vi "Ponk.vi"() -> ()   [LabVIEW 2022 SP3]
uses:
  <vilib>/Utility/miscctls.llb/LVPositionTypeDef.ctl
panel:
  out "BarPosition 2":T1
  out "Bar 2":bool
  out "Top":bool
  out "exit?":bool
  in  "STOP":bool
  out "BarPosition":T1
  out "BallPosition":T1
  out "Step":T1
  out "Bar":bool
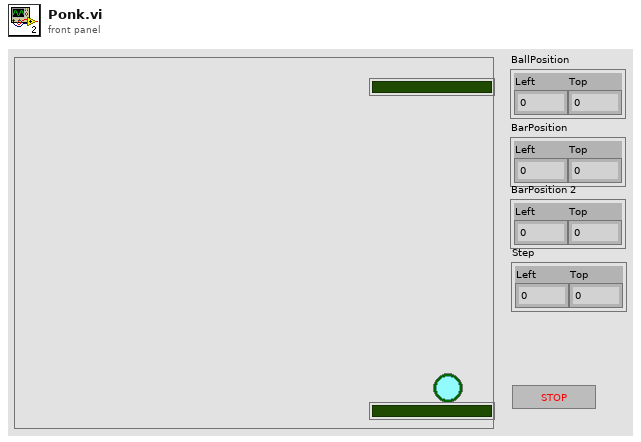
[diagram p1: front panel]
types:
  T1 = typedef "LVPositionTypeDef.ctl" = cluster{"Left":i32, "Top":i32}
  T2 = cluster{"BallPosition":T1, "Step":T1, "Score":i32, "BarPosition":T1, "BarPosition_2":T1}
  T3 = typedef "LVBoundsTypeDef.ctl" = cluster{"Width":u32, "Height":u32}
  T4 = typedef "eventvkey.ctl" = enum16{"ASCII", "Enter", "Return", "Shift", "Ctrl", "Alt", "Cmd", "Opt", "Caps", "NumLock", "Clear", "Break", "Up", "Down", "Left", "Right", "Insert", "Delete", "Home", "End", "PageUp", "PageDown", "Escape", "Help", "Pause", "ScrollLock", "F1", "F2", "F3", "F4", "F5", "F6", "F7", "F8", "F9", "F10", "F11", "F12", "F13", "F14", "F15", "F16", "F17", "F18", "F19", "F20", "F21", "F22", "F23", "F24", "Play", "VolumeUp", "VolumeDown", "Mute", "Two Byte Char"}
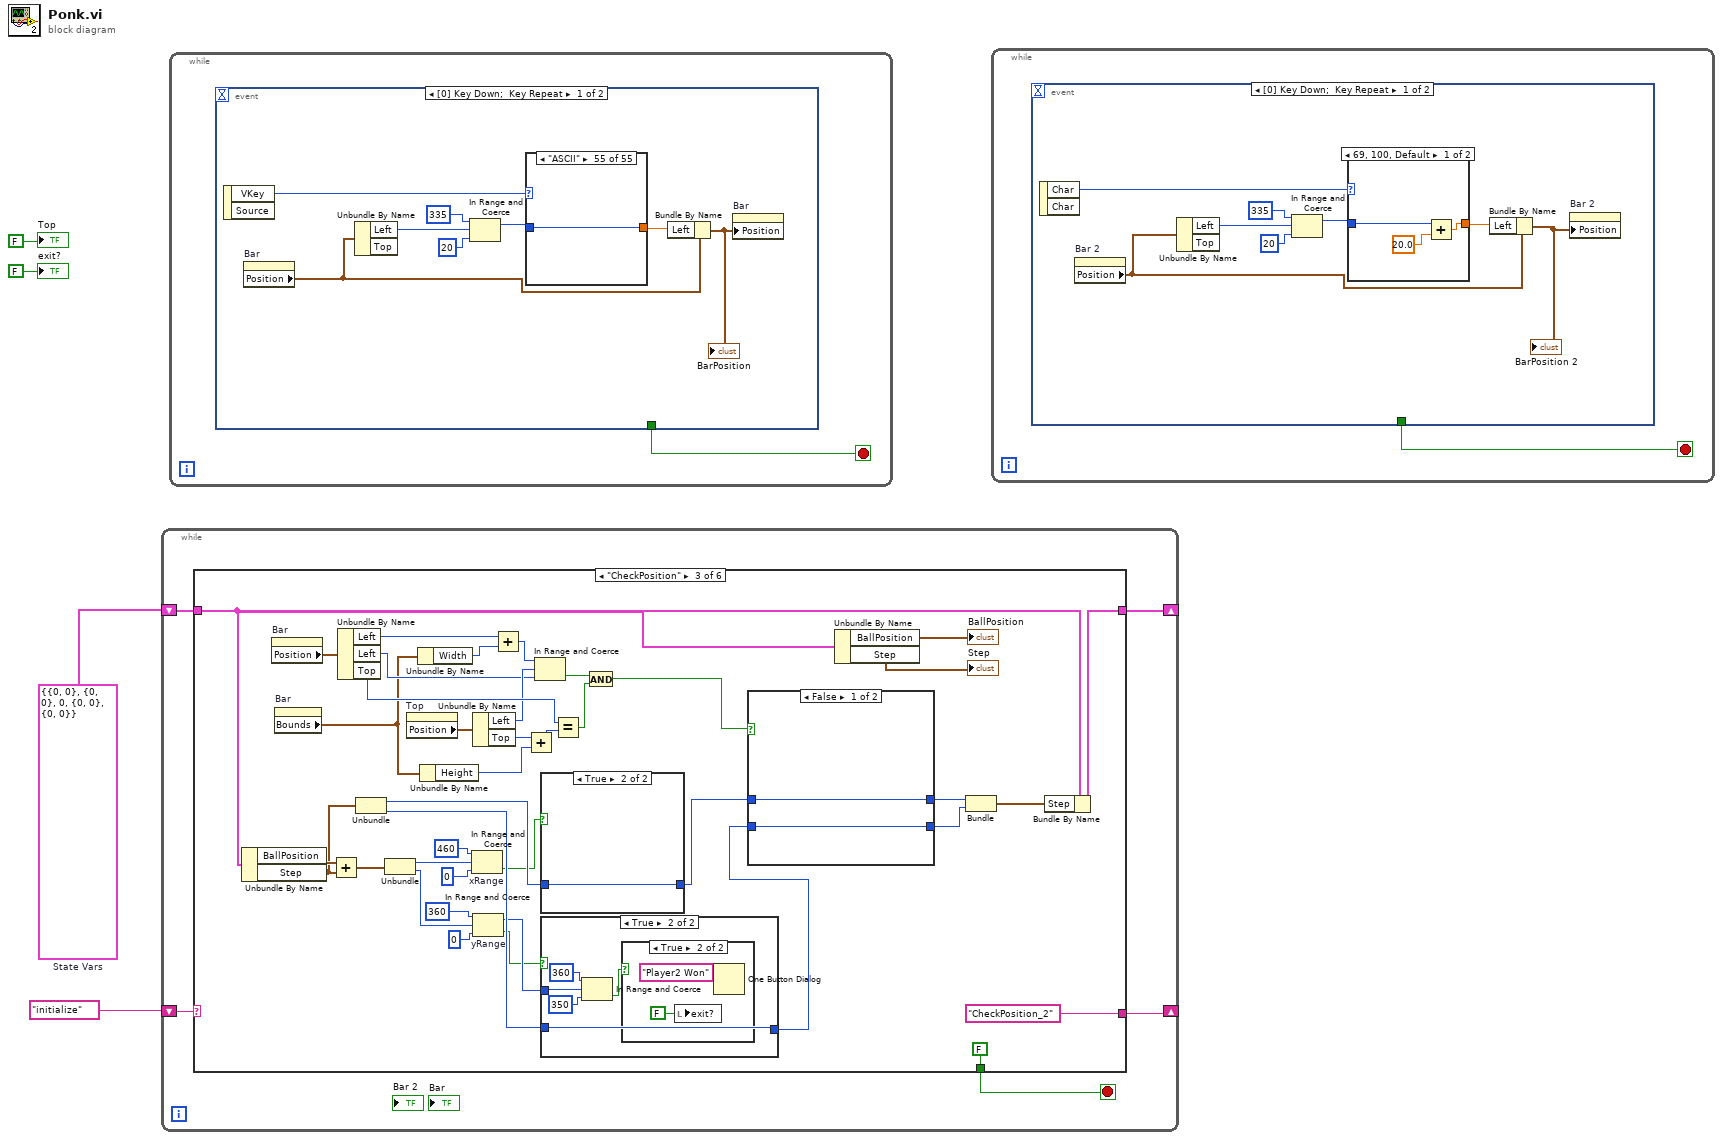
[diagram p0: block diagram]
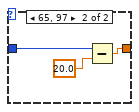
[diagram p2: hidden frame]
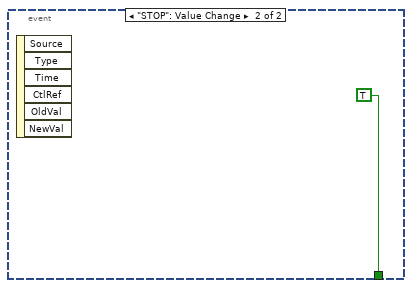
[diagram p3: hidden frame]
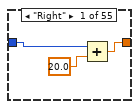
[diagram p4: hidden frame]
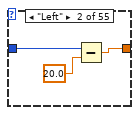
[diagram p5: hidden frame]
diagram:
  w3 = T2 {"BallPosition"={"Left"=0, "Top"=0}, "Step"={"Left"=0, "Top"=0}, "Score"=0, "BarPosition"={"Left"=0, "Top"=0}, "BarPosition_2"={"Left"=0, "Top"=0}}  # State Vars
  n1 = while {
    shift-right: [w7] -> _
    shift-left: "initialize" -> [w6]
    shift-right: [w8] -> _
    shift-left: w3 -> [w9]
    stop <- w5 stop-if-true
    n2 = case shown="\"CheckPosition\"" w6 {
      selector: w6 -> [w11 _ _ _ _ _]
      tunnel: w9 -> [w12 w30 w43 w99 w144 w147]
      tunnel: [w12 w29 w60 w115 w144 w151] -> w8
      tunnel: [w11 "UpdateBallPosition" "CheckPosition_2" "Stop" "UpdateBallPosition" "CheckPosition"] -> w7
      tunnel: [FALSE ("STOP") FALSE ("STOP") FALSE ("STOP") FALSE ("STOP") "STOP" FALSE ("STOP")] -> w5
      frame "False", Default {
      }
      frame "Initialize" {
        n3 = property on="Bar" class="Bool (strict)"() -> ("Bounds"=w23:T3)  [unwired: 2 in, 2 out]
        n4 = Unbundle By Name(w23) -> ("Width"=w22:u32)
        n5 = property on="Bar" class="Bool (strict)"() -> ("Position"=w24:T1)  [unwired: 2 in, 2 out]
        n6 = Unbundle By Name(w24) -> ("Left"=w21:i32, "Top"=w19:i32)
        n7 = Divide(x=w22, y=u32 2) -> (x/y=w20:dbl)
        n8 = Add(x=w20, y=w21) -> (x+y=w18:dbl)
        n9 = Add(x=w19, y=-30) -> (x+y=w17:i32)
        n10 = Bundle(w18, w17) -> (w14:cluster{dbl, i32})  [unwired: 1 in]
        n11 = Bundle By Name(cluster=w30, "BallPosition"=w14, "Step"=T1 {"Left"=1, "Top"=1}, "BarPosition"=T1 {"Left"=0, "Top"=0}, "BarPosition_2"=T1 {"Left"=0, "Top"=0} ("BarPosition")) -> (w29:T2)
      }
      frame "CheckPosition" {
        n12 = Unbundle By Name(w43) -> ("BallPosition"=w70:T1, "Step"=w50:T1)
        n13 = property on="Bar" class="Bool (strict)"() -> ("Position"=w53:T1)  [unwired: 2 in, 2 out]
        n14 = property on="Bar" class="Bool (strict)"() -> ("Bounds"=w34:T3)  [unwired: 2 in, 2 out]
        n15 = Add(x=w70, y=w50) -> (x+y=w69:T1)
        n16 = Unbundle By Name(w53) -> ("Left"=w54:i32, "Left"=w38:i32, "Top"=w40:i32)
        n17 = Unbundle(w50) -> ("Left"=w62:i32, "Top"=w61:i32)
        n18 = Unbundle(w69) -> ("Left"=w68:i32, "Top"=w63:i32)
        n19 = property on="Top" class="Bool (strict)"() -> ("Position"=w52:T1)  [unwired: 2 in, 2 out]
        n20 = Unbundle By Name(w34) -> ("Width"=w35:u32)
        n21 = Unbundle By Name(w34) -> ("Height"=w33:u32)
        n22 = In Range and Coerce "xRange"(upper limit=460, x=w68, lower limit=0) -> (In Range?=w51:bool)  [unwired: 1 out]
        n23 = Unbundle By Name(w52) -> ("Left"=w39:i32, "Top"=w37:i32)
        n24 = In Range and Coerce "yRange"(upper limit=360, x=w63, lower limit=0) -> (coerced(x)=w58:i32, In Range?=w32:bool)
        n25 = Add(x=w54, y=w35) -> (x+y=w55:u32)
        n26 = Add(x=w37, y=w33) -> (x+y=w36:u32)
        n27 = In Range and Coerce(upper limit=w55, x=w39, lower limit=w38) -> (In Range?=w57:bool)  [unwired: 1 out]
        n28 = case shown="True" w51 {
          tunnel: [w85 w87] -> w48
          tunnel: w62 -> [w86 w87]
          frame False {
            n29 = Negate(x=w86) -> (-x=w85:i32)
          }
          frame True {
          }
        }
        n30 = case shown="True" w32 {
          tunnel: [w77 w82] -> w49
          tunnel: w61 -> [w76 w82]
          tunnel: w58 -> [_ w79]
          frame False {
            n31 = Negate(x=w76) -> (-x=w77:i32)
          }
          frame True {
            n32 = In Range and Coerce(upper limit=360, x=w79, lower limit=350) -> (In Range?=w78:bool)  [unwired: 1 out]
            n33 = case shown="True" w78 {
              frame False {
              }
              frame True {
                n34 = local write "exit?"(FALSE ("exit?")) -> ()
                n35 = One Button Dialog(message="Player2 Won") -> ()  [unwired: 1 in, 1 out]
              }
            }
          }
        }
        n36 = Equal?(x=w40, y=w36) -> (x = y?=w56:bool)
        n37 = And(x=w57, y=w56) -> (x .and. y?=w44:bool)
        n38 = case shown="False" w44 {
          tunnel: w49 -> [w71 w75]
          tunnel: w48 -> [w72 w73]
          tunnel: [w72 w73] -> w46
          tunnel: [w71 w74] -> w47
          frame False {
          }
          frame True {
            n39 = Negate(x=w75) -> (-x=w74:i32)
          }
        }
        n40 = Unbundle By Name(w43) -> ("BallPosition"=→"BallPosition":T1, "Step"=→"Step":T1)
        n41 = Bundle("Left"=w46, "Top"=w47) -> (w45:cluster{"Left":i32, "Top":i32})  [unwired: 1 in]
        n42 = Bundle By Name(cluster=w43, "Step"=w45) -> (w60:T2)
      }
      frame "CheckPosition_2" {
        n43 = Unbundle By Name(w99) -> ("BallPosition"=w125:T1, "Step"=w106:T1)
        n44 = property on="Bar 2" class="Bool (strict)"() -> ("Position"=w92:T1)  [unwired: 2 in, 2 out]
        n45 = property on="Bar 2" class="Bool (strict)"() -> ("Bounds"=w91:T3)  [unwired: 2 in, 2 out]
        n46 = Unbundle By Name(w91) -> ("Width"=w90:u32, "Height"=w93:u32)
        n47 = Add(x=w125, y=w106) -> (x+y=w124:T1)
        n48 = Unbundle By Name(w92) -> ("Left"=w109:i32, "Left"=w96:i32, "Top"=w98:i32)
        n49 = Unbundle(w106) -> ("Left"=w117:i32, "Top"=w116:i32)
        n50 = Unbundle(w124) -> ("Left"=w123:i32, "Top"=w118:i32)
        n51 = property on="Top" class="Bool (strict)"() -> ("Position"=w108:T1)  [unwired: 2 in, 2 out]
        n52 = In Range and Coerce "xRange"(upper limit=460, x=w123, lower limit=0) -> (In Range?=w107:bool)  [unwired: 1 out]
        n53 = Unbundle By Name(w108) -> ("Left"=w97:i32, "Top"=w95:i32)
        n54 = In Range and Coerce "yRange"(upper limit=360, x=w118, lower limit=0) -> (coerced(x)=w113:i32, In Range?=w89:bool)
        n55 = Add(x=w109, y=w90) -> (x+y=w110:u32)
        n56 = Subtract(x=w95, y=w93) -> (x-y=w94:u32)
        n57 = In Range and Coerce(upper limit=w110, x=w97, lower limit=w96) -> (In Range?=w112:bool)  [unwired: 1 out]
        n58 = case shown="True" w107 {
          tunnel: [w140 w142] -> w104
          tunnel: w117 -> [w141 w142]
          frame False {
            n59 = Negate(x=w141) -> (-x=w140:i32)
          }
          frame True {
          }
        }
        n60 = case shown="True" w89 {
          tunnel: [w132 w137] -> w105
          tunnel: w116 -> [w131 w137]
          tunnel: w113 -> [_ w134]
          frame False {
            n61 = Negate(x=w131) -> (-x=w132:i32)
          }
          frame True {
            n62 = In Range and Coerce(upper limit=12, x=w134, lower limit=0) -> (In Range?=w133:bool)  [unwired: 1 out]
            n63 = case shown="True" w133 {
              frame False {
              }
              frame True {
                n64 = local write "exit?"(TRUE ("exit?")) -> ()
                n65 = One Button Dialog(message="Player1 Won") -> ()  [unwired: 1 in, 1 out]
              }
            }
          }
        }
        n66 = Equal?(x=w98, y=w94) -> (x = y?=w111:bool)
        n67 = And(x=w112, y=w111) -> (x .and. y?=w100:bool)
        n68 = case shown="True" w100 {
          tunnel: w105 -> [w126 w130]
          tunnel: w104 -> [w127 w128]
          tunnel: [w127 w128] -> w102
          tunnel: [w126 w129] -> w103
          frame False {
          }
          frame True {
            n69 = Negate(x=w130) -> (-x=w129:i32)
          }
        }
        n70 = Bundle("Left"=w102, "Top"=w103) -> (w101:cluster{"Left":i32, "Top":i32})  [unwired: 1 in]
        n71 = Bundle By Name(cluster=w99, "Step"=w101) -> (w115:T2)
      }
      frame "Stop" {
      }
      frame "UpdateBallPosition" {
        n72 = Unbundle By Name(w147) -> ("BallPosition"=w152:T1, "Step"=w153:T1)
        n73 = Add(x=w152, y=w153) -> (x+y=w150:T1)
        n74 = Bundle By Name(cluster=w147, "BallPosition"=w150) -> (w151:T2)
        n75 = property on="Top" class="Bool (strict)"("Position"=w150) -> ()  [unwired: 2 in, 2 out]
        n76 = Wait (ms)(milliseconds to wait=u32 7) -> ()  [unwired: 1 out]
      }
    }
  }
  n77 = while {
    stop <- w154 stop-if-true
    n78 = event shown="[0] Key Down;  Key Repeat" {
      selector: _ -> [_ _]
      dyn-events: _ -> [_ _]
      timeout: _ -> [_ _]
      tunnel: [_ TRUE] -> w154
      event Key Down; Key Repeat {
        n79 = event-data() -> ("VKey"=w155:T4)  [unwired: 1 in, 1 out]
        n80 = property on="Bar" class="Bool (strict)"() -> ("Position"=w161:T1)  [unwired: 2 in, 2 out]
        n81 = Unbundle By Name(w161) -> ("Left"=w158:i32)  [unwired: 1 out]
        n82 = In Range and Coerce(upper limit=335, x=w158, lower limit=20) -> (coerced(x)=w159:i32)  [unwired: 1 out]
        n83 = case shown="\"ASCII\"" w155 {
          tunnel: w159 -> [w164 w166 w169 w170 w171 w172 w173 w174 w175 w176 w177 w178 w179 w180 w181 w182 w183 w184 w185 w186 w187 w188 w189 w190 w191 w192 w193 w194 w195 w196 w197 w198 w199 w200 w201 w202 w203 w204 w205 w206 w207 w208 w209 w210 w211 w212 w213 w214 w215 w216 w217 w218 w219 w220 w221]
          tunnel: [w163 w167 w169 w170 w171 w172 w173 w174 w175 w176 w177 w178 w179 w180 w181 w182 w183 w184 w185 w186 w187 w188 w189 w190 w191 w192 w193 w194 w195 w196 w197 w198 w199 w200 w201 w202 w203 w204 w205 w206 w207 w208 w209 w210 w211 w212 w213 w214 w215 w216 w217 w218 w219 w220 w221] -> w162
          frame "Right" {
            n84 = Add(x=w164, y=20.0) -> (x+y=w163:dbl)
          }
          frame "Left" {
            n85 = Subtract(x=w166, y=20.0) -> (x-y=w167:dbl)
          }
          frame "F16" {
          }
          frame "F17" {
          }
          frame "F18" {
          }
          frame "F19" {
          }
          frame "F20" {
          }
          frame "F21" {
          }
          frame "F22" {
          }
          frame "F23" {
          }
          frame "F24" {
          }
          frame "Play" {
          }
          frame "VolumeUp" {
          }
          frame "VolumeDown" {
          }
          frame "Mute" {
          }
          frame "Two Byte Char" {
          }
          frame "Insert" {
          }
          frame "Delete" {
          }
          frame "Home" {
          }
          frame "End" {
          }
          frame "PageUp" {
          }
          frame "PageDown" {
          }
          frame "Escape" {
          }
          frame "Help" {
          }
          frame "Pause" {
          }
          frame "ScrollLock" {
          }
          frame "F1" {
          }
          frame "F2" {
          }
          frame "F3" {
          }
          frame "F4" {
          }
          frame "F5" {
          }
          frame "F6" {
          }
          frame "F7" {
          }
          frame "F8" {
          }
          frame "F9" {
          }
          frame "F10" {
          }
          frame "F11" {
          }
          frame "F12" {
          }
          frame "F13" {
          }
          frame "F14" {
          }
          frame "F15" {
          }
          frame "Down" {
          }
          frame "Up" {
          }
          frame "Break" {
          }
          frame "Clear" {
          }
          frame "NumLock" {
          }
          frame "Caps" {
          }
          frame "Opt" {
          }
          frame "Cmd" {
          }
          frame "Alt" {
          }
          frame "Ctrl" {
          }
          frame "Shift" {
          }
          frame "Return" {
          }
          frame "Enter" {
          }
          frame "ASCII" {
          }
        }
        n86 = Bundle By Name(cluster=w161, "Left"=w162) -> (w160:T1)
        "BarPosition" <- w160
        n87 = property on="Bar" class="Bool (strict)"("Position"=w160) -> ()  [unwired: 2 in, 2 out]
      }
      event "STOP": Value Change {
        n88 = event-data() -> ()  [unwired: 1 in, 4 out]
      }
    }
  }
  n89 = while {
    stop <- w223 stop-if-true
    n90 = event shown="[0] Key Down;  Key Repeat" {
      selector: _ -> [_ _]
      dyn-events: _ -> [_ _]
      timeout: _ -> [_ _]
      tunnel: [_ TRUE] -> w223
      event Key Down; Key Repeat {
        n91 = event-data() -> ("Char"=w226:i16)  [unwired: 1 in, 1 out]
        n92 = property on="Bar 2" class="Bool (strict)"() -> ("Position"=w225:T1)  [unwired: 2 in, 2 out]
        n93 = Unbundle By Name(w225) -> ("Left"=w229:i32)  [unwired: 1 out]
        n94 = In Range and Coerce(upper limit=335, x=w229, lower limit=20) -> (coerced(x)=w230:i32)  [unwired: 1 out]
        n95 = case shown="69, 100, Default" w226 {
          tunnel: w230 -> [w233 w236]
          tunnel: [w232 w235] -> w231
          frame 69, 100, Default {
            n96 = Add(x=w233, y=20.0) -> (x+y=w232:dbl)
          }
          frame 65, 97 {
            n97 = Subtract(x=w236, y=20.0) -> (x-y=w235:dbl)
          }
        }
        n98 = Bundle By Name(cluster=w225, "Left"=w231) -> (w224:T1)
        "BarPosition 2" <- w224
        n99 = property on="Bar 2" class="Bool (strict)"("Position"=w224) -> ()  [unwired: 2 in, 2 out]
      }
      event "STOP": Value Change {
        n100 = event-data() -> ()  [unwired: 1 in, 6 out]
      }
    }
  }
  "exit?" <- FALSE ("exit?")
  "Top" <- FALSE ("Top")
